vi "2022_day06.vi"() -> ()   [LabVIEW 2021]
panel:
  out "Results":cluster{"Found?":bool, "Msg Position":i32}[](array[cluster])
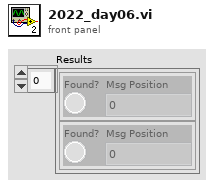
[diagram p1: front panel]
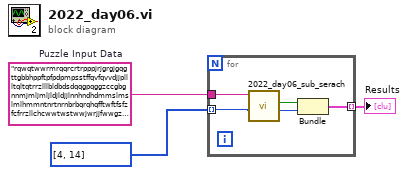
[diagram p0: block diagram]
diagram:
  w3 = "rqwqtwwrmrqqrcrtrpppjrjgrgjgqgttgbbhppftpfpdpmpsstffqvfqvvdjjpllltqltqtrrzlllbldbdsdqqgpqggzccgbgnnmjmljmljldjldjjlnnhndhdmmslmslmlhmmntnrtnrnbrbqrqhqfftwftfsfzfcfrrzllchcwwtwstwwjwrjjfwwgzwzqzpzhzqhqbhqhssltsszhsszdssrwssdppjcpjjrwjwnwjnnzjjhsjhsjsjvvtffffqfflglwglgbgpbgbgghfghfhdfhdfhfssqppvlvslltwwhwvwpwgggnpnnmqnntqnnlhhdbhdbbtvvcrrcgrrdrvrjvvlmlnmndnmnrncnznsnsqnsswrwzwmwzzbpbhphqhpqpbpqpjpjvpvwpvwppdvdhdccqbccfncctrcrjcjjdsdhdnhhwpwlwwbmbhmbhhpzhhccvffqqnsqqmnnspnnpfpzppspgsppgbbdwbbdcchfhgfhfllljtllnjlnlddvcdvdqvvqwqppprtpthtthqqfbqqpfpzfpfcfsscrsccbgbngbbgdbbpgpqqlmqlmmgffqqqsbqbtblbwb..."  # Puzzle Input Data
  n1 = for {
    tunnel: w3 -> [w8]
    tunnel: i32[] [4, 14] -> [w5] mode=indexing
    tunnel: [w4] -> w1 mode=indexing
    n2 = call "2022_day06_sub_serach.vi"("# of consecutive unique characters"=w5, "Puzzle Input Data"=w8) -> ("Msg Position"=w7:i32, "Found?"=w6:bool)  [unwired: 8 in]
    n3 = Bundle("Found?"=w6, "Msg Position"=w7) -> (w4:cluster{"Found?":bool, "Msg Position":i32})  [unwired: 1 in]
  }
  "Results" <- w1
